vi "Calculate Driving Direction of Tank1.vi"() -> ()   [LabVIEW 2012]
doc: "Calculates the velocity vector of the robot required to avoid obstacles, based on the scanned data."
uses:
  <vilib>/imath/engines/lvmath2/RunTimeEngine/ErrorHandling/NIMS_Finalize Error.vi
  <vilib>/imath/engines/lvmath2/RunTimeEngine/BuiltInFunctions/abs/NIMS_abs(signed).vi
  <instcachedir>/0/NIMS_abs(signed)_C4FCB8E6058B49B797C7C8D53CA5F6EC.lvgen/NIMS_abs(signed)_C4FCB8E6058B49B797C7C8D53CA5F6EC_000.vi
  <vilib>/imath/engines/lvmath2/RunTimeEngine/VariableToken/NIMS_VariableToken_CondDefined.vi
  <instcachedir>/0/NIMS_VariableToken_CondDefined_295AAB8C64C949DA8EA45AB7820AF759.lvgen/NIMS_VariableToken_CondDefined_295AAB8C64C949DA8EA45AB7820AF759_003.vi
  <vilib>/imathl/engines/lvmath/Functions/Error Handling/Create Error.vi
  <instcachedir>/0/NIMS_VariableToken_CondDefined_295AAB8C64C949DA8EA45AB7820AF759.lvgen/NIMS_VariableToken_CondDefined_295AAB8C64C949DA8EA45AB7820AF759_004.vi
  <vilib>/imath/engines/lvmath/Functions/Error Handling/MergeErrorsWrapper.vi
  <vilib>/imath/engines/lvmath2/RunTimeEngine/NodeEndStatement/NIMS_NodeEndStatement_Output.vi
  <instcachedir>/0/NIMS_NodeEndStatement_Output_53EC0D466D134D7ABD903AC30B43404B.lvgen/NIMS_NodeEndStatement_Output_53EC0D466D134D7ABD903AC30B43404B_001.vi
  <instcachedir>/0/NIMS_NodeEndStatement_Output_53EC0D466D134D7ABD903AC30B43404B.lvgen/NIMS_NodeEndStatement_Output_53EC0D466D134D7ABD903AC30B43404B_013.vi
panel:
  in  "dir1":dbl
  in  "angle":dbl
  in  "max angular velocity (rad/s)":dbl=1.0
  in  "max reverse velocity (m/s)":dbl
  in  "kaiguan":bool
  out "angle 2":dbl
  in  "find":bool
  out "t":dbl
  out "appended array":dbl[](array[numeric])
  out "error out":errorcluster
  in  "error in (no error)":errorcluster
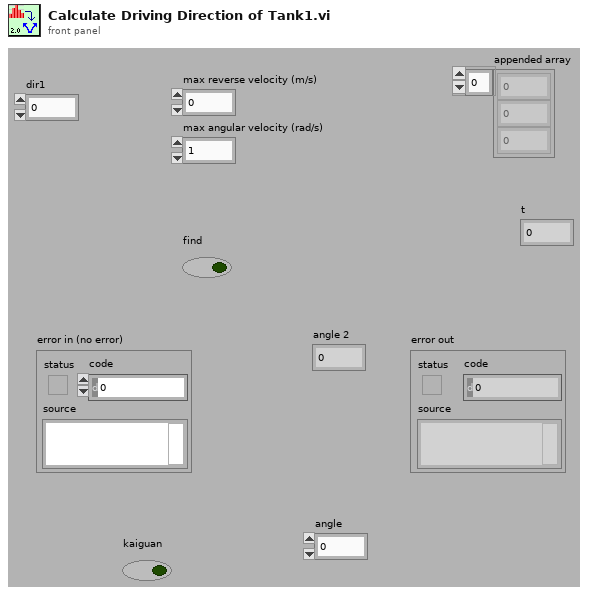
[diagram p1: front panel]
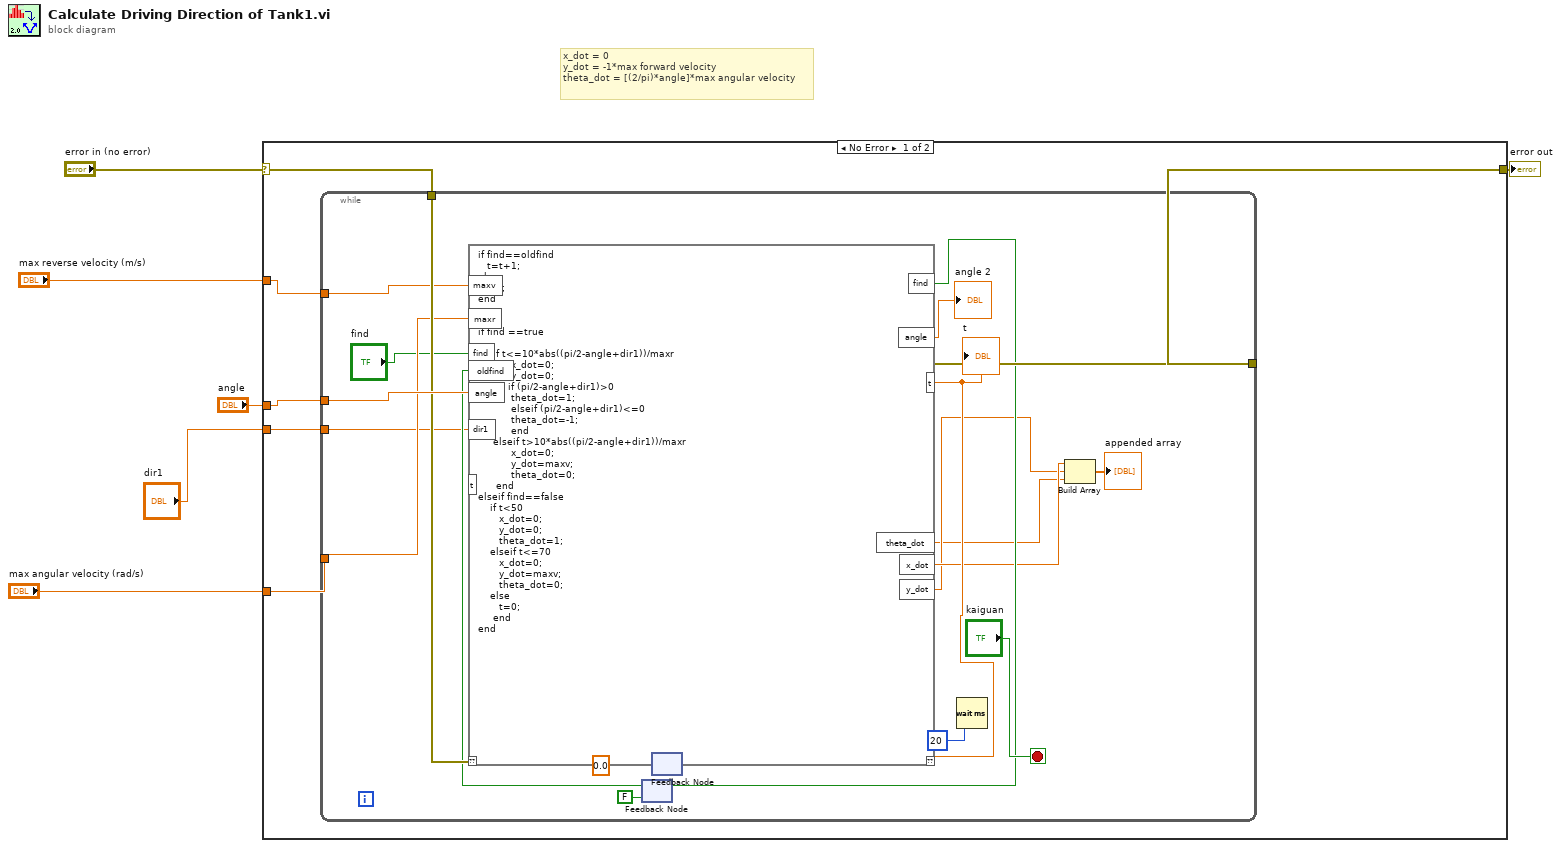
[diagram p0: block diagram]
diagram:
  # "x_dot = 0\ny_dot = -1*max forward velocity\ntheta_dot = [(2/pi)*angle]*max angular velocity"
  n1 = case shown="No Error" "error in (no error)" {
    selector: "error in (no error)" -> [w9 w382]
    tunnel: [w8 w382] -> w5
    tunnel: "max reverse velocity (m/s)" -> [w12 _]
    tunnel: "max angular velocity (rad/s)" -> [w11 _]
    tunnel: "angle" -> [w10 _]
    tunnel: "dir1" -> [w7 _]
    frame No Error {
      n2 = while {
        tunnel: w12 -> [w29]
        tunnel: w11 -> [w28]
        tunnel: w10 -> [w32]
        tunnel: w9 -> [w31]
        tunnel: [w30] -> w8
        tunnel: w7 -> [w18]
        stop <- "kaiguan" stop-if-true
        n3 = feedback #1(FALSE ("find")) -> (w21:bool)
        n4 = feedback #2(0.0 ("t")) -> (w23:dbl)
        n5 = mathscript code="if find==oldfind\n   t=t+1;\nelse\n  t=0;\nend\n\n\nif find ==true\n     \n     if t<=10*abs((pi/2-angle+dir1))/maxr\n           x_dot=0;\n           y_dot=0; \n          if (pi/2-angle+dir1)>0\n           theta_dot=1;\n           elseif (pi/2-angle+dir1)<=0\n           theta_dot=-1;\n           end\n     elseif t>10*abs((pi/2-angle+dir1))/maxr\n           x_dot=0;\n           y_dot=maxv;\n           theta_dot=0;\n      end\nelseif find==false\n    if t<50\n       x_dot=0;\n       y_dot=0;\n       theta_dot=1;\n    elseif t<=70\n       x_dot=0;\n       y_dot=maxv;\n       theta_dot=0;\n    else\n       t=0;\n     end\nend"("??"=w31, "maxv"=w29, "maxr"=w28, "find"="find", "angle"=w32, "dir1"=w18, "t"=w23, "oldfind"=w21) -> ("??"=w30:errorcluster, "theta_dot"=w14:dbl, "y_dot"=w15:dbl, "t"=w24:dbl, "angle"=→"angle 2":dbl, "find"=w22:bool, "x_dot"=w16:dbl)
        "t" <- w24
        n6 = feedback-in #1(w22) -> ()
        n7 = feedback-in #2(w24) -> ()
        n8 = Wait (ms)(milliseconds to wait=u32 20) -> ()  [unwired: 1 out]
        n9 = Build Array(w16, w15, w14) -> (→"appended array":dbl[])
      }
    }
    frame Error {
    }
  }
  "error out" <- w5
